vi "Read Log Session.vi"(8 "error in (no error)":errorcluster, 11 "Network Actor in":refnum<class "Network Actor.lvclass">) -> (0 "error out":errorcluster, 2 "Session Handle":T1, 3 "Network Actor out":refnum<class "Network Actor.lvclass">)   [LabVIEW 2014, in "Network Actor Library.lvlib" / "Network Actor.lvclass"]
uses:
  Network Actor.lvclass
  <userlib>/_Session Fwk/Typedefs/Session Handle.ctl
  <userlib>/_Session Fwk/Session - Root.lvclass
  Network Actor.lvclass/Network Actor.ctl
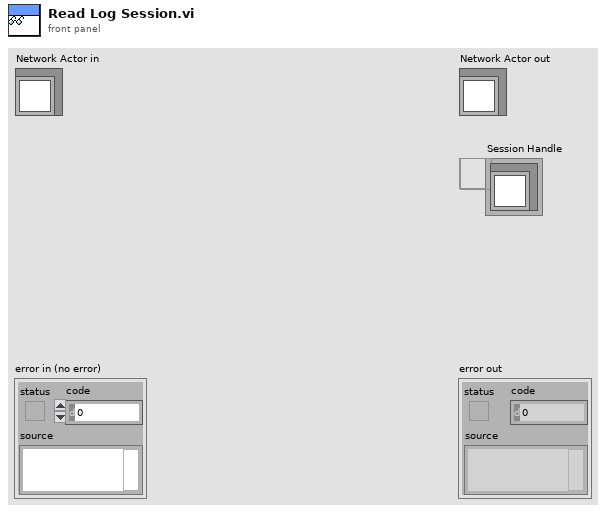
[diagram p1: front panel]
types:
  T1 = typedef "Session - Root.lvclass/Session Handle.ctl" = refnum<data-value>
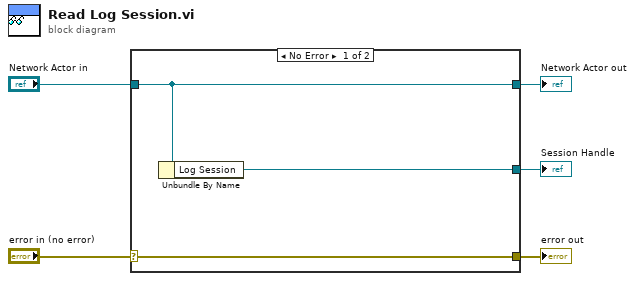
[diagram p0: block diagram]
diagram:
  n1 = case shown="No Error" "error in (no error)" {
    selector: "error in (no error)" -> [w8 w9]
    tunnel: [w8 w9] -> w4
    tunnel: [w7 w10] -> w2
    tunnel: "Network Actor in" -> [w7 w10]
    tunnel: [w6 _] -> w1
    frame No Error {
      n2 = Unbundle By Name(w7) -> ("Log Session"=w6:T1)
    }
    frame Error {
    }
  }
  "error out" <- w4
  "Network Actor out" <- w2
  "Session Handle" <- w1
